vi "MainInit Queue.vi"(8 "error in":errorcluster) -> (0 "error out":errorcluster)   [LabVIEW 2022 SP3]
uses:
  Type Def/MainStates Cluster.ctl
  Type Def/MainStates.ctl
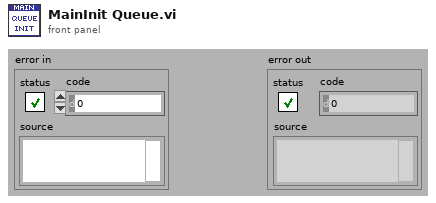
[diagram p1: front panel]
types:
  T1 = typedef "MainStates Cluster.ctl" = cluster{"States":T2, "Data":variant}
  T2 = typedef "MainStates.ctl" = enum16{"Open Ports", "Close Ports", "Main", "Settings", "Voltaje", "Probe", "Lenguaje", "Callibration", "Exit", "Voltage Test", "Test 2", "End test"}
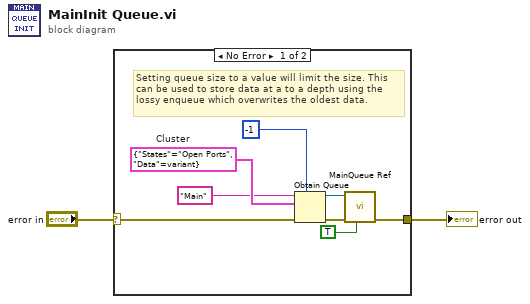
[diagram p0: block diagram]
diagram:
  n1 = case shown="No Error" "error in" {
    selector: "error in" -> [w8 w11]
    tunnel: [w9 w11] -> w1
    frame No Error {
      w6 = T1 {"States"=enum."Open Ports", "Data"=variant}  # Cluster
      # "Setting queue size to a value will limit the size. This can be used to store data at a to a depth using the\nlossy enqueue which overwrites the oldest data."
      n2 = Obtain Queue(max queue size (-1, unlimited)=-1, name (unnamed)="Main", element data type=w6, error in (no error)=w8) -> (queue out=w4:refnum<queue>, error out=w7:errorcluster)  [unwired: 1 in, 1 out]
      n3 = call "MainQueue Ref.vi"("Write:T/Read:(F)"=TRUE ("Write:T/Read:F"), "error in"=w7, "queue in"=w4) -> ("error out"=w9:errorcluster)  [unwired: 7 in, 1 out]
    }
    frame Error {
    }
  }
  "error out" <- w1
